vi "Halfwave Fit.vi"(4 "Offset":dbl, 6 "Ignore Offset":bool, 8 "Sample Rate":i32, 9 "Phase (deg)":dbl format="%#_13g", 10 "Stimulus\nFrequency":dbl=nan, 11 "Data in":dbl[](array[numeric])) -> (2 "Best Fit":dbl[](array[numeric]), 3 "Coefficients":T1 {"Freq" format="%#.2f"; "Offset" format="%.3f"; "Gain" format="%.2f"; "Phase" format="%.1f"})   [LabVIEW 2016, in "Halfwave Sinusoidal Fit.lvclass"]
uses:
  Halfwave Sinusoidal Fit.lvclass
  gain and phase/Typedef - Sinusoidal Fit Coefficients.ctl
  <vilib>/Analysis/NI_AALPro.lvlib
  Abstract Fit/Abstract Fit.lvclass
panel:
  out "Waveform Graph":dbl[][](graph)
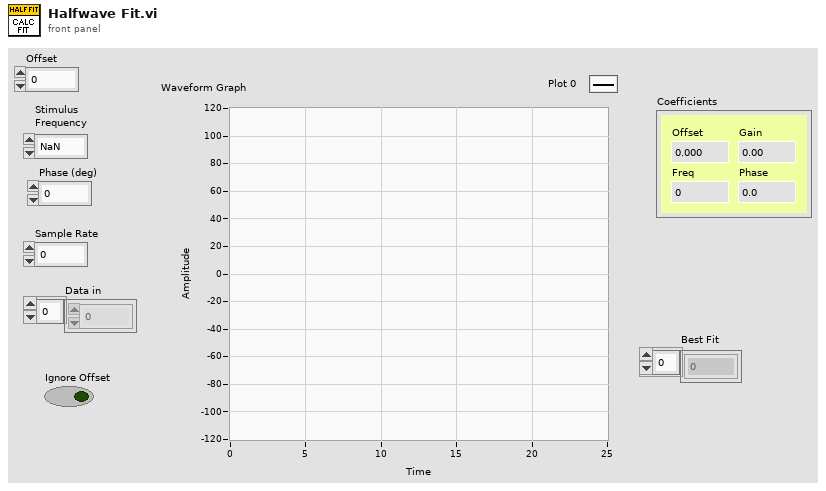
[diagram p1: front panel]
types:
  T1 = typedef "Typedef - Sinusoidal Fit Coefficients.ctl" = cluster{"Offset":dbl, "Gain":dbl, "Phase":dbl, "Freq":dbl}
  T2 = cluster{dbl, dbl, "Phase (deg)":dbl, "Fundamental frequency":dbl}
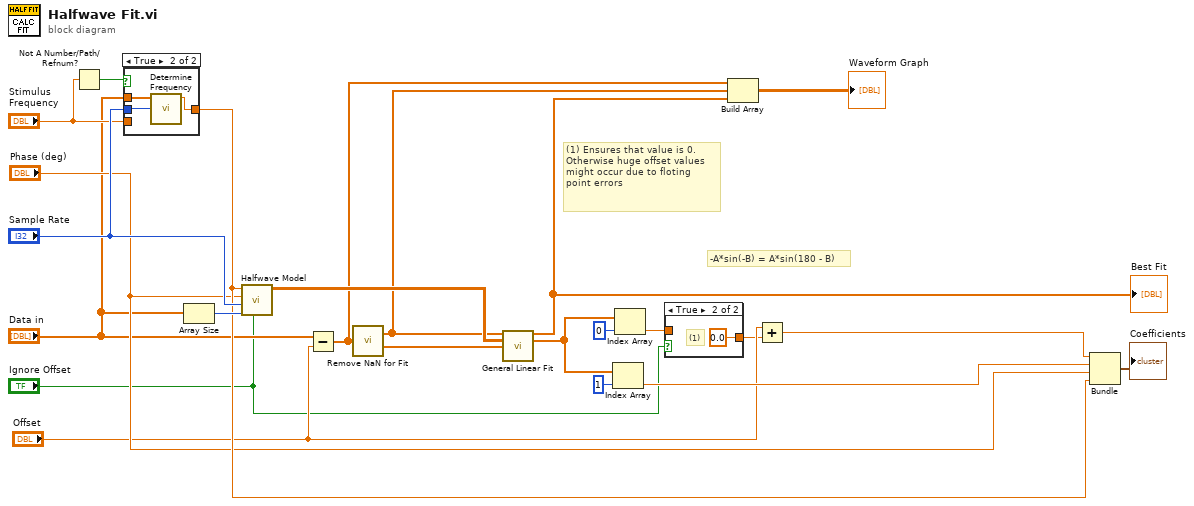
[diagram p0: block diagram]
diagram:
  # "(1) Ensures that value is 0. Otherwise huge offset values might occur due to floting point errors"
  # "-A*sin(-B) = A*sin(180 - B)"
  n1 = Not A Number/Path/Refnum?(number/path/refnum="Stimulus\nFrequency") -> (NaN/Path/Refnum?=w16:bool)
  n2 = case shown="True" w16 {
    tunnel: [w24 w26] -> w17
    tunnel: "Stimulus\nFrequency" -> [w24 _]
    tunnel: "Data in" -> [_ w27]
    tunnel: "Sample Rate" -> [_ w25]
    frame False {
    }
    frame True {
      n3 = call "Determine Frequency.vi"("Sample Rate"=w25, "Signal (in)"=w27) -> ("Fundamental frequency"=w26:dbl)  [unwired: 5 in]
    }
  }
  n4 = Array Size(array="Data in") -> (size(s)=w22:i32)
  n5 = call "Halfwave Model.vi"("Ignore Offset"="Ignore Offset", "Length"=w22, "Sample Rate"="Sample Rate", "Phase (deg)"="Phase (deg)", "Frequency"=w17) -> ("Array"=w12:dbl[][])  [unwired: 6 in]
  n6 = Subtract(x="Data in", y="Offset") -> (x-y=w6:dbl[])
  n7 = call "Remove NaN for Fit.vi"("Data in"=w6) -> ("Weight out"=w11:dbl[], "Data out"=w10:dbl[])  [unwired: 2 in]
  n8 = call <vilib>:"General Linear Fit.vi"("Y"=w10, "H"=w12, "Weight"=w11) -> ("Best Fit"=w20:dbl[], "Coefficients"=w9:dbl[])  [unwired: 7 in, 4 out]
  "Best Fit" <- w20
  n9 = Index Array(array=w9, index=1 ("Index")) -> (element=w13:dbl)
  n10 = Index Array(array=w9, index=0) -> (element=w2:dbl)
  n11 = case shown="True" "Ignore Offset" {
    tunnel: w2 -> [w28 _]
    tunnel: [w28 0.0] -> w1
    frame False {
    }
    frame True {
      # "(1)"
    }
  }
  n12 = Build Array(w6, w10, w20) -> (→"Waveform Graph":dbl[][])
  n13 = Add(x="Offset", y=w1) -> (x+y=w7:dbl)
  n14 = Bundle(w7, w13, "Phase (deg)"="Phase (deg)", "Fundamental frequency"=w17) -> (→"Coefficients":T2)  [unwired: 1 in]
